vi "输入数据解析.vi"(0 "单个参数补充":dbl, 1 "从板号":dbl=1.0, 2 "主板二维码":string="BNET01", 3 "从板二维码":string="BNET01", 5 "主板引用":refnum<vi>, 7 "从板引用":refnum<vi>, 9 "主板选项":string="三级故障阀值", 11 "枚举":enum16{"主板", "从板"}(ring), 12 "快换":bool caption="快换写入") -> (4 "输出数组":dbl[][](array[numeric]), 6 "数组长度":dbl[](array[numeric]), 8 "循环次数":i32, 10 "命令":u32, 14 "名称":string[](array[string]), 15 "命令序号":u32[](array[numeric]))   [LabVIEW 2013] (continued)
                n3829 = Build Array(w9934) -> (w9935:dbl[])
              }
              frame 15 {
                # "极柱温度过高"
                n3830 = disable-structure shown="启用" {
                  disable-tunnel: w9945 -> [w9951 _]
                  disable-tunnel: [w9947 255 ("高字节1")] -> w9943
                  frame Disabled {
                    n3831 = Unbundle By Name(w9951) -> ("极柱温度过高"=w9950:dbl)
                    n3832 = call "输入分辨率计算-EV05.vi"("1字节?"=TRUE, "数值"=w9950, "偏移量"=-40.0, "分辨率"=1.0) -> ("高字节1"=w9947:dbl)  [unwired: 1 in, 6 out]
                  }
                  frame Enabled {
                  }
                }
                n3833 = Build Array(w9943) -> (w9944:i32[])
              }
              frame 16 {
                # "SOH过低"
                n3834 = disable-structure shown="启用" {
                  disable-tunnel: [w9968 w9976] -> w9955
                  disable-tunnel: w9954 -> [w9965 _]
                  disable-tunnel: [w9957 w9976] -> w9953
                  frame Disabled {
                    n3835 = Unbundle By Name(w9965) -> ("SOH过低"=w9964:dbl)
                    n3836 = call "输入分辨率计算-EV05.vi"("1字节?"=FALSE, "数值"=w9964, "偏移量"=0.0, "分辨率"=0.1) -> ("低字节"=w9966:dbl, "高字节1"=w9967:dbl)  [unwired: 1 in, 5 out]
                    n3837 = call "二进制解析-8.6.vi"("索引"=4, "数值"=w9967) -> ("低位子数组"=w9970:i32[])  [unwired: 3 out]
                    n3838 = call "二进制解析-8.6.vi"("索引"=4, "数值"=w9966) -> ("低位子数组"=w9959:i32[], "高位子数组"=w9969:i32[])  [unwired: 2 out]
                    n3839 = call "二进制解析-8.6.vi"("索引"=4, "数值"=0) -> ("低位子数组"=w9960:i32[])  [unwired: 3 out]
                    n3840 = Insert Into Array(array=w9970, new element=w9969) -> (w9963:i32[])  [unwired: 1 in]
                    n3841 = Insert Into Array(array=w9959, new element=w9960) -> (w9958:i32[])  [unwired: 1 in]
                    n3842 = call "数值二进制转十进制-8.6.vi"("子数组"=w9963) -> ("十进制数值"=w9968:i32)  [unwired: 4 out]
                    n3843 = call "数值二进制转十进制-8.6.vi"("子数组"=w9958) -> ("十进制数值"=w9957:i32)  [unwired: 4 out]
                  }
                  frame Enabled {
                    w9976 = 255 ("高字节1")
                  }
                }
                n3844 = Build Array(w9955, w9953) -> (w9956:i32[])
              }
            }
            n3845 = Insert Into Array(array=w9761, new element=w9762) -> (w9760:dbl[])  [unwired: 1 in]
          }
          n3846 = Build Array(w9757) -> (w9756:dbl[][])
          n3847 = Build Array("三级故障阀值") -> (w9747:string[])
        }
        frame "极柱温度过高" {
          n3848 = Unbundle By Name(w9982) -> ("一级故障"=w9983:refnum<vi>)
          n3849 = property class="Clust (严格)"(reference=w9983) -> ("Value"=w9981:T4)  [unwired: 1 in, 2 out]
          n3850 = for {
            N: 17 -> [_]
            tunnel: w9981 -> [w9993]
            shift-right: [w9990] -> w9987
            shift-left: dbl[] [] -> [w9991]
            i -> [w9994]
            n3851 = case shown="13" w9994 {
              tunnel: w9993 -> [w9995 w10006 w10017 w10027 w10037 w10047 w10059 w10071 w10083 w10095 w10107 w10119 w10133 w10154 w10166 w10175 w10184]
              tunnel: [w9996 w10007 w10018 w10028 w10038 w10049 w10061 w10073 w10085 w10097 w10109 w10120 w10142 w10157 w10165 w10174 w10186] -> w9992
              frame 0, Default {
                # "总电压过高"
                n3852 = disable-structure shown="启用" {
                  disable-tunnel: [w10002 w10005] -> w9998
                  disable-tunnel: [w10001 w10005] -> w9997
                  disable-tunnel: w9995 -> [w10000 _]
                  frame Disabled {
                    n3853 = Unbundle By Name(w10000) -> ("总电压过高"=w9999:dbl)
                    n3854 = call "输入分辨率计算-EV05.vi"("1字节?"=FALSE, "数值"=w9999, "分辨率"=0.1) -> ("低字节"=w10002:dbl, "高字节1"=w10001:dbl)  [unwired: 2 in, 5 out]
                  }
                  frame Enabled {
                    w10005 = 255 ("高字节1")
                  }
                }
                n3855 = Build Array(w9997, w9998) -> (w9996:i32[])
              }
              frame 1 {
                # "总电压过低"
                n3856 = disable-structure shown="启用" {
                  disable-tunnel: [w10013 w10016] -> w10009
                  disable-tunnel: [w10012 w10016] -> w10008
                  disable-tunnel: w10006 -> [w10011 _]
                  frame Disabled {
                    n3857 = Unbundle By Name(w10011) -> ("总电压过低"=w10010:dbl)
                    n3858 = call "输入分辨率计算-EV05.vi"("1字节?"=FALSE, "数值"=w10010, "分辨率"=0.1) -> ("低字节"=w10013:dbl, "高字节1"=w10012:dbl)  [unwired: 2 in, 5 out]
                  }
                  frame Enabled {
                    w10016 = 255 ("高字节1")
                  }
                }
                n3859 = Build Array(w10008, w10009) -> (w10007:i32[])
              }
              frame 2 {
                # "温度过高"
                n3860 = disable-structure shown="启用" {
                  disable-tunnel: [w10023 255 ("高字节1")] -> w10019
                  disable-tunnel: w10017 -> [w10021 _]
                  frame Disabled {
                    n3861 = Unbundle By Name(w10021) -> ("温度过高"=w10020:dbl)
                    n3862 = call "输入分辨率计算-EV05.vi"("1字节?"=TRUE, "数值"=w10020, "偏移量"=-40.0, "分辨率"=1.0) -> ("高字节1"=w10023:dbl)  [unwired: 1 in, 6 out]
                  }
                  frame Enabled {
                  }
                }
                n3863 = Build Array(w10019) -> (w10018:i32[])
              }
              frame 3 {
                # "温度过低"
                n3864 = disable-structure shown="启用" {
                  disable-tunnel: [w10033 255 ("高字节1")] -> w10029
                  disable-tunnel: w10027 -> [w10031 _]
                  frame Disabled {
                    n3865 = Unbundle By Name(w10031) -> ("温度过低"=w10030:dbl)
                    n3866 = call "输入分辨率计算-EV05.vi"("1字节?"=TRUE, "数值"=w10030, "偏移量"=-40.0, "分辨率"=1.0) -> ("高字节1"=w10033:dbl)  [unwired: 1 in, 6 out]
                  }
                  frame Enabled {
                  }
                }
                n3867 = Build Array(w10029) -> (w10028:i32[])
              }
              frame 4 {
                # "整组温度不均衡"
                n3868 = disable-structure shown="启用" {
                  disable-tunnel: [w10043 255 ("高字节1")] -> w10039
                  disable-tunnel: w10037 -> [w10041 _]
                  frame Disabled {
                    n3869 = Unbundle By Name(w10041) -> ("整组温度不均衡"=w10040:dbl)
                    n3870 = call "输入分辨率计算-EV05.vi"("1字节?"=TRUE, "数值"=w10040, "偏移量"=0.0, "分辨率"=1.0) -> ("高字节1"=w10043:dbl)  [unwired: 1 in, 6 out]
                  }
                  frame Enabled {
                  }
                }
                n3871 = Build Array(w10039) -> (w10038:i32[])
              }
              frame 5 {
                # "单组电压不均衡"
                n3872 = disable-structure shown="启用" {
                  disable-tunnel: [w10055 w10058] -> w10050
                  disable-tunnel: [w10053 w10058] -> w10048
                  disable-tunnel: w10047 -> [w10052 _]
                  frame Disabled {
                    n3873 = Unbundle By Name(w10052) -> ("单组电压不均衡"=w10051:dbl)
                    n3874 = call "输入分辨率计算-EV05.vi"("1字节?"=FALSE, "数值"=w10051, "偏移量"=0.0, "分辨率"=0.001) -> ("低字节"=w10053:dbl, "高字节1"=w10055:dbl)  [unwired: 1 in, 5 out]
                  }
                  frame Enabled {
                    w10058 = 255 ("高字节1")
                  }
                }
                n3875 = Build Array(w10050, w10048) -> (w10049:i32[])
              }
              frame 6 {
                # "整组电压不均衡"
                n3876 = disable-structure shown="启用" {
                  disable-tunnel: [w10067 w10070] -> w10062
                  disable-tunnel: [w10065 w10070] -> w10060
                  disable-tunnel: w10059 -> [w10064 _]
                  frame Disabled {
                    n3877 = Unbundle By Name(w10064) -> ("整组电压不均衡"=w10063:dbl)
                    n3878 = call "输入分辨率计算-EV05.vi"("1字节?"=FALSE, "数值"=w10063, "偏移量"=0.0, "分辨率"=0.001) -> ("低字节"=w10065:dbl, "高字节1"=w10067:dbl)  [unwired: 1 in, 5 out]
                  }
                  frame Enabled {
                    w10070 = 255 ("高字节1")
                  }
                }
                n3879 = Build Array(w10062, w10060) -> (w10061:i32[])
              }
              frame 7 {
                # "单体电压过高"
                n3880 = disable-structure shown="启用" {
                  disable-tunnel: [w10079 w10082] -> w10074
                  disable-tunnel: [w10077 w10082] -> w10072
                  disable-tunnel: w10071 -> [w10076 _]
                  frame Disabled {
                    n3881 = Unbundle By Name(w10076) -> ("单体电压过高"=w10075:dbl)
                    n3882 = call "输入分辨率计算-EV05.vi"("1字节?"=FALSE, "数值"=w10075, "偏移量"=0.0, "分辨率"=0.001) -> ("低字节"=w10077:dbl, "高字节1"=w10079:dbl)  [unwired: 1 in, 5 out]
                  }
                  frame Enabled {
                    w10082 = 255 ("高字节1")
                  }
                }
                n3883 = Build Array(w10074, w10072) -> (w10073:i32[])
              }
              frame 8 {
                # "单体电压过低"
                n3884 = disable-structure shown="启用" {
                  disable-tunnel: [w10091 w10094] -> w10086
                  disable-tunnel: [w10089 w10094] -> w10084
                  disable-tunnel: w10083 -> [w10088 _]
                  frame Disabled {
                    n3885 = Unbundle By Name(w10088) -> ("单体电压过低"=w10087:dbl)
                    n3886 = call "输入分辨率计算-EV05.vi"("1字节?"=FALSE, "数值"=w10087, "偏移量"=0.0, "分辨率"=0.001) -> ("低字节"=w10089:dbl, "高字节1"=w10091:dbl)  [unwired: 1 in, 5 out]
                  }
                  frame Enabled {
                    w10094 = 255 ("高字节1")
                  }
                }
                n3887 = Build Array(w10086, w10084) -> (w10085:i32[])
              }
              frame 9 {
                # "充电电流过高"
                n3888 = disable-structure shown="启用" {
                  disable-tunnel: [w10103 w10106] -> w10098
                  disable-tunnel: [w10101 w10106] -> w10096
                  disable-tunnel: w10095 -> [w10100 _]
                  frame Disabled {
                    n3889 = Unbundle By Name(w10100) -> ("充电电流过高"=w10099:dbl)
                    n3890 = call "输入分辨率计算-EV05.vi"("1字节?"=FALSE, "数值"=w10099, "偏移量"=-3000.0, "分辨率"=0.1) -> ("低字节"=w10101:dbl, "高字节1"=w10103:dbl)  [unwired: 1 in, 5 out]
                  }
                  frame Enabled {
                    w10106 = 255 ("高字节1")
                  }
                }
                n3891 = Build Array(w10098, w10096) -> (w10097:i32[])
              }
              frame 10 {
                # "放电电流过高"
                n3892 = disable-structure shown="启用" {
                  disable-tunnel: [w10115 w10118] -> w10110
                  disable-tunnel: [w10113 w10118] -> w10108
                  disable-tunnel: w10107 -> [w10112 _]
                  frame Disabled {
                    n3893 = Unbundle By Name(w10112) -> ("放电电流过高"=w10111:dbl)
                    n3894 = call "输入分辨率计算-EV05.vi"("1字节?"=FALSE, "数值"=w10111, "偏移量"=-3000.0, "分辨率"=0.1) -> ("低字节"=w10113:dbl, "高字节1"=w10115:dbl)  [unwired: 1 in, 5 out]
                  }
                  frame Enabled {
                    w10118 = 255 ("高字节1")
                  }
                }
                n3895 = Build Array(w10110, w10108) -> (w10109:i32[])
              }
              frame 11 {
                # "单组温度不均衡"
                n3896 = disable-structure shown="启用" {
                  disable-tunnel: [w10125 255 ("高字节1")] -> w10121
                  disable-tunnel: w10119 -> [w10123 _]
                  frame Disabled {
                    n3897 = Unbundle By Name(w10123) -> ("单组温度不均衡"=w10122:dbl)
                    n3898 = call "输入分辨率计算-EV05.vi"("1字节?"=TRUE, "数值"=w10122, "偏移量"=0.0, "分辨率"=1.0) -> ("高字节1"=w10125:dbl)  [unwired: 1 in, 6 out]
                  }
                  frame Enabled {
                  }
                }
                n3899 = Build Array(w10121) -> (w10120:i32[])
              }
              frame 12 {
                # "SOC过高"
                n3900 = Unbundle By Name(w10133) -> ("SOC过高"=w10132:dbl)
                n3901 = call "输入分辨率计算-EV05.vi"("1字节?"=FALSE, "数值"=w10132, "偏移量"=0.0, "分辨率"=0.1) -> ("低字节"=w10134:dbl, "高字节1"=w10135:dbl)  [unwired: 1 in, 5 out]
                n3902 = call "二进制解析-8.6.vi"("索引"=4, "数值"=w10135) -> ("低位子数组"=w10138:i32[])  [unwired: 3 out]
                n3903 = call "二进制解析-8.6.vi"("索引"=4, "数值"=w10134) -> ("低位子数组"=w10130:i32[], "高位子数组"=w10137:i32[])  [unwired: 2 out]
                n3904 = Insert Into Array(array=w10138, new element=w10137) -> (w10136:i32[])  [unwired: 1 in]
                n3905 = call "数值二进制转十进制-8.6.vi"("子数组"=w10136) -> ("十进制数值"=w10131:i32)  [unwired: 4 out]
                n3906 = disable-structure shown="启用" {
                  disable-tunnel: w10131 -> [w10146 _]
                  disable-tunnel: [w10146 255 ("高字节1")] -> w10129
                  disable-tunnel: w10130 -> [w10145 _]
                  disable-tunnel: [w10145 i32[] [] ("低位子数组 29")] -> _
                  frame Disabled {
                  }
                  frame Enabled {
                  }
                }
                n3907 = Build Array(w10129, w10129) -> (w10142:i32[])
              }
              frame 13 {
                # "SOC过低"
                n3908 = Unbundle By Name(w10154) -> ("SOC过低"=w10153:dbl)
                n3909 = call "输入分辨率计算-EV05.vi"("1字节?"=FALSE, "数值"=w10153, "偏移量"=0.0, "分辨率"=0.1) -> ("低字节"=w10151:dbl, "高字节1"=w10152:dbl)  [unwired: 1 in, 5 out]
                n3910 = call "二进制解析-8.6.vi"("索引"=4, "数值"=w10152) -> ("低位子数组"=w10150:i32[])  [unwired: 3 out]
                n3911 = disable-structure shown="启用" {
                  disable-tunnel: w10151 -> [w10161 _]
                  disable-tunnel: [w10161 255 ("高字节1")] -> w10149
                  disable-tunnel: w10150 -> [w10160 _]
                  disable-tunnel: [w10160 i32[] [] ("低位子数组")] -> _
                  frame Disabled {
                    (unwired) i32[] [] ("低位子数组 4")
                  }
                  frame Enabled {
                  }
                }
                n3912 = Build Array(w10149, w10149) -> (w10157:i32[])
              }
              frame 14 {
                # "内阻过大"
                n3913 = disable-structure shown="启用" {
                  disable-tunnel: w10166 -> [w10171 _]
                  disable-tunnel: [w10167 255 ("高字节1")] -> w10164
                  frame Disabled {
                    n3914 = Unbundle By Name(w10171) -> ("内阻过大"=w10170:dbl)
                    n3915 = call "输入分辨率计算-EV05.vi"("1字节?"=TRUE, "数值"=w10170, "分辨率"=0.1) -> ("高字节1"=w10167:dbl)  [unwired: 2 in, 6 out]
                  }
                  frame Enabled {
                  }
                }
                n3916 = Build Array(w10164) -> (w10165:i32[])
              }
              frame 15 {
                # "极柱温度过高"
                n3917 = disable-structure shown="启用" {
                  disable-tunnel: w10175 -> [w10181 _]
                  disable-tunnel: [w10177 255 ("高字节1")] -> w10173
                  frame Enabled {
                    n3918 = Unbundle By Name(w10181) -> ("极柱温度过高"=w10180:dbl)
                    n3919 = call "输入分辨率计算-EV05.vi"("1字节?"=TRUE, "数值"=w10180, "偏移量"=-40.0, "分辨率"=1.0) -> ("高字节1"=w10177:dbl)  [unwired: 1 in, 6 out]
                  }
                  frame Disabled {
                  }
                }
                n3920 = Build Array(w10173) -> (w10174:dbl[])
              }
              frame 16 {
                # "SOH过低"
                n3921 = disable-structure shown="启用" {
                  disable-tunnel: [w10198 w10206] -> w10185
                  disable-tunnel: w10184 -> [w10195 _]
                  disable-tunnel: [w10187 w10206] -> w10183
                  frame Disabled {
                    n3922 = Unbundle By Name(w10195) -> ("SOH过低"=w10194:dbl)
                    n3923 = call "输入分辨率计算-EV05.vi"("1字节?"=FALSE, "数值"=w10194, "偏移量"=0.0, "分辨率"=0.1) -> ("低字节"=w10196:dbl, "高字节1"=w10197:dbl)  [unwired: 1 in, 5 out]
                    n3924 = call "二进制解析-8.6.vi"("索引"=4, "数值"=w10197) -> ("低位子数组"=w10200:i32[])  [unwired: 3 out]
                    n3925 = call "二进制解析-8.6.vi"("索引"=4, "数值"=w10196) -> ("低位子数组"=w10189:i32[], "高位子数组"=w10199:i32[])  [unwired: 2 out]
                    n3926 = call "二进制解析-8.6.vi"("索引"=4, "数值"=0) -> ("低位子数组"=w10190:i32[])  [unwired: 3 out]
                    n3927 = Insert Into Array(array=w10200, new element=w10199) -> (w10193:i32[])  [unwired: 1 in]
                    n3928 = Insert Into Array(array=w10189, new element=w10190) -> (w10188:i32[])  [unwired: 1 in]
                    n3929 = call "数值二进制转十进制-8.6.vi"("子数组"=w10193) -> ("十进制数值"=w10198:i32)  [unwired: 4 out]
                    n3930 = call "数值二进制转十进制-8.6.vi"("子数组"=w10188) -> ("十进制数值"=w10187:i32)  [unwired: 4 out]
                  }
                  frame Enabled {
                    w10206 = 255 ("高字节1")
                  }
                }
                n3931 = Build Array(w10185, w10183) -> (w10186:i32[])
              }
            }
            n3932 = Insert Into Array(array=w9991, new element=w9992) -> (w9990:dbl[])  [unwired: 1 in]
          }
          n3933 = Build Array(w9987) -> (w9986:dbl[][])
          n3934 = Build Array("一级故障阀值") -> (w9977:string[])
        }
        frame "极柱温度过高(2)" {
          n3935 = Unbundle By Name(w10212) -> ("一级故障 2"=w10213:refnum<vi>)
          n3936 = property class="Clust (严格)"(reference=w10213) -> ("Value"=w10211:T4)  [unwired: 1 in, 2 out]
          n3937 = for {
            N: 17 -> [_]
            tunnel: w10211 -> [w10223]
            shift-right: [w10220] -> w10217
            shift-left: dbl[] [] -> [w10221]
            i -> [w10224]
            n3938 = case shown="13" w10224 {
              tunnel: w10223 -> [w10225 w10236 w10247 w10257 w10267 w10277 w10289 w10301 w10313 w10325 w10337 w10349 w10363 w10384 w10396 w10405 w10414]
              tunnel: [w10226 w10237 w10248 w10258 w10268 w10279 w10291 w10303 w10315 w10327 w10339 w10350 w10372 w10387 w10395 w10404 w10416] -> w10222
              frame 0, Default {
                # "总电压过高"
                n3939 = disable-structure shown="启用" {
                  disable-tunnel: [w10232 w10235] -> w10228
                  disable-tunnel: [w10231 w10235] -> w10227
                  disable-tunnel: w10225 -> [w10230 _]
                  frame Disabled {
                    n3940 = Unbundle By Name(w10230) -> ("总电压过高"=w10229:dbl)
                    n3941 = call "输入分辨率计算-EV05.vi"("1字节?"=FALSE, "数值"=w10229, "分辨率"=0.1) -> ("低字节"=w10232:dbl, "高字节1"=w10231:dbl)  [unwired: 2 in, 5 out]
                  }
                  frame Enabled {
                    w10235 = 255 ("高字节1")
                  }
                }
                n3942 = Build Array(w10227, w10228) -> (w10226:i32[])
              }
              frame 1 {
                # "总电压过低"
                n3943 = disable-structure shown="启用" {
                  disable-tunnel: [w10243 w10246] -> w10239
                  disable-tunnel: [w10242 w10246] -> w10238
                  disable-tunnel: w10236 -> [w10241 _]
                  frame Disabled {
                    n3944 = Unbundle By Name(w10241) -> ("总电压过低"=w10240:dbl)
                    n3945 = call "输入分辨率计算-EV05.vi"("1字节?"=FALSE, "数值"=w10240, "分辨率"=0.1) -> ("低字节"=w10243:dbl, "高字节1"=w10242:dbl)  [unwired: 2 in, 5 out]
                  }
                  frame Enabled {
                    w10246 = 255 ("高字节1")
                  }
                }
                n3946 = Build Array(w10238, w10239) -> (w10237:i32[])
              }
              frame 2 {
                # "温度过高"
                n3947 = disable-structure shown="启用" {
                  disable-tunnel: [w10253 255 ("高字节1")] -> w10249
                  disable-tunnel: w10247 -> [w10251 _]
                  frame Disabled {
                    n3948 = Unbundle By Name(w10251) -> ("温度过高"=w10250:dbl)
                    n3949 = call "输入分辨率计算-EV05.vi"("1字节?"=TRUE, "数值"=w10250, "偏移量"=-40.0, "分辨率"=1.0) -> ("高字节1"=w10253:dbl)  [unwired: 1 in, 6 out]
                  }
                  frame Enabled {
                  }
                }
                n3950 = Build Array(w10249) -> (w10248:i32[])
              }
              frame 3 {
                # "温度过低"
                n3951 = disable-structure shown="启用" {
                  disable-tunnel: [w10263 255 ("高字节1")] -> w10259
                  disable-tunnel: w10257 -> [w10261 _]
                  frame Disabled {
                    n3952 = Unbundle By Name(w10261) -> ("温度过低"=w10260:dbl)
                    n3953 = call "输入分辨率计算-EV05.vi"("1字节?"=TRUE, "数值"=w10260, "偏移量"=-40.0, "分辨率"=1.0) -> ("高字节1"=w10263:dbl)  [unwired: 1 in, 6 out]
                  }
                  frame Enabled {
                  }
                }
                n3954 = Build Array(w10259) -> (w10258:i32[])
              }
              frame 4 {
                # "整组温度不均衡"
                n3955 = disable-structure shown="启用" {
                  disable-tunnel: [w10273 255 ("高字节1")] -> w10269
                  disable-tunnel: w10267 -> [w10271 _]
                  frame Disabled {
                    n3956 = Unbundle By Name(w10271) -> ("整组温度不均衡"=w10270:dbl)
                    n3957 = call "输入分辨率计算-EV05.vi"("1字节?"=TRUE, "数值"=w10270, "偏移量"=0.0, "分辨率"=1.0) -> ("高字节1"=w10273:dbl)  [unwired: 1 in, 6 out]
                  }
                  frame Enabled {
                  }
                }
                n3958 = Build Array(w10269) -> (w10268:i32[])
              }
              frame 5 {
                # "单组电压不均衡"
                n3959 = disable-structure shown="启用" {
                  disable-tunnel: [w10285 w10288] -> w10280
                  disable-tunnel: [w10283 w10288] -> w10278
                  disable-tunnel: w10277 -> [w10282 _]
                  frame Disabled {
                    n3960 = Unbundle By Name(w10282) -> ("单组电压不均衡"=w10281:dbl)
                    n3961 = call "输入分辨率计算-EV05.vi"("1字节?"=FALSE, "数值"=w10281, "偏移量"=0.0, "分辨率"=0.001) -> ("低字节"=w10283:dbl, "高字节1"=w10285:dbl)  [unwired: 1 in, 5 out]
                  }
                  frame Enabled {
                    w10288 = 255 ("高字节1")
                  }
                }
                n3962 = Build Array(w10280, w10278) -> (w10279:i32[])
              }
              frame 6 {
                # "整组电压不均衡"
                n3963 = disable-structure shown="启用" {
                  disable-tunnel: [w10297 w10300] -> w10292
                  disable-tunnel: [w10295 w10300] -> w10290
                  disable-tunnel: w10289 -> [w10294 _]
                  frame Disabled {
                    n3964 = Unbundle By Name(w10294) -> ("整组电压不均衡"=w10293:dbl)
                    n3965 = call "输入分辨率计算-EV05.vi"("1字节?"=FALSE, "数值"=w10293, "偏移量"=0.0, "分辨率"=0.001) -> ("低字节"=w10295:dbl, "高字节1"=w10297:dbl)  [unwired: 1 in, 5 out]
                  }
                  frame Enabled {
                    w10300 = 255 ("高字节1")
                  }
                }
                n3966 = Build Array(w10292, w10290) -> (w10291:i32[])
              }
              frame 7 {
                # "单体电压过高"
                n3967 = disable-structure shown="启用" {
                  disable-tunnel: [w10309 w10312] -> w10304
                  disable-tunnel: [w10307 w10312] -> w10302
                  disable-tunnel: w10301 -> [w10306 _]
                  frame Disabled {
                    n3968 = Unbundle By Name(w10306) -> ("单体电压过高"=w10305:dbl)
                    n3969 = call "输入分辨率计算-EV05.vi"("1字节?"=FALSE, "数值"=w10305, "偏移量"=0.0, "分辨率"=0.001) -> ("低字节"=w10307:dbl, "高字节1"=w10309:dbl)  [unwired: 1 in, 5 out]
                  }
                  frame Enabled {
                    w10312 = 255 ("高字节1")
                  }
                }
                n3970 = Build Array(w10304, w10302) -> (w10303:i32[])
              }
              frame 8 {
                # "单体电压过低"
                n3971 = disable-structure shown="启用" {
                  disable-tunnel: [w10321 w10324] -> w10316
                  disable-tunnel: [w10319 w10324] -> w10314
                  disable-tunnel: w10313 -> [w10318 _]
                  frame Disabled {
                    n3972 = Unbundle By Name(w10318) -> ("单体电压过低"=w10317:dbl)
                    n3973 = call "输入分辨率计算-EV05.vi"("1字节?"=FALSE, "数值"=w10317, "偏移量"=0.0, "分辨率"=0.001) -> ("低字节"=w10319:dbl, "高字节1"=w10321:dbl)  [unwired: 1 in, 5 out]
                  }
                  frame Enabled {
                    w10324 = 255 ("高字节1")
                  }
                }
                n3974 = Build Array(w10316, w10314) -> (w10315:i32[])
              }
              frame 9 {
                # "充电电流过高"
                n3975 = disable-structure shown="启用" {
                  disable-tunnel: [w10333 w10336] -> w10328
                  disable-tunnel: [w10331 w10336] -> w10326
                  disable-tunnel: w10325 -> [w10330 _]
                  frame Disabled {
                    n3976 = Unbundle By Name(w10330) -> ("充电电流过高"=w10329:dbl)
                    n3977 = call "输入分辨率计算-EV05.vi"("1字节?"=FALSE, "数值"=w10329, "偏移量"=-3000.0, "分辨率"=0.1) -> ("低字节"=w10331:dbl, "高字节1"=w10333:dbl)  [unwired: 1 in, 5 out]
                  }
                  frame Enabled {
                    w10336 = 255 ("高字节1")
                  }
                }
                n3978 = Build Array(w10328, w10326) -> (w10327:i32[])
              }
              frame 10 {
                # "放电电流过高"
                n3979 = disable-structure shown="启用" {
                  disable-tunnel: [w10345 w10348] -> w10340
                  disable-tunnel: [w10343 w10348] -> w10338
                  disable-tunnel: w10337 -> [w10342 _]
                  frame Disabled {
                    n3980 = Unbundle By Name(w10342) -> ("放电电流过高"=w10341:dbl)
                    n3981 = call "输入分辨率计算-EV05.vi"("1字节?"=FALSE, "数值"=w10341, "偏移量"=-3000.0, "分辨率"=0.1) -> ("低字节"=w10343:dbl, "高字节1"=w10345:dbl)  [unwired: 1 in, 5 out]
                  }
                  frame Enabled {
                    w10348 = 255 ("高字节1")
                  }
                }
                n3982 = Build Array(w10340, w10338) -> (w10339:i32[])
              }
              frame 11 {
                # "单组温度不均衡"
                n3983 = disable-structure shown="启用" {
                  disable-tunnel: [w10355 255 ("高字节1")] -> w10351
                  disable-tunnel: w10349 -> [w10353 _]
                  frame Disabled {
                    n3984 = Unbundle By Name(w10353) -> ("单组温度不均衡"=w10352:dbl)
                    n3985 = call "输入分辨率计算-EV05.vi"("1字节?"=TRUE, "数值"=w10352, "偏移量"=0.0, "分辨率"=1.0) -> ("高字节1"=w10355:dbl)  [unwired: 1 in, 6 out]
                  }
                  frame Enabled {
                  }
                }
                n3986 = Build Array(w10351) -> (w10350:i32[])
              }
              frame 12 {
                # "SOC过高"
                n3987 = Unbundle By Name(w10363) -> ("SOC过高"=w10362:dbl)
                n3988 = call "输入分辨率计算-EV05.vi"("1字节?"=FALSE, "数值"=w10362, "偏移量"=0.0, "分辨率"=0.1) -> ("低字节"=w10364:dbl, "高字节1"=w10365:dbl)  [unwired: 1 in, 5 out]
                n3989 = call "二进制解析-8.6.vi"("索引"=4, "数值"=w10365) -> ("低位子数组"=w10368:i32[])  [unwired: 3 out]
                n3990 = call "二进制解析-8.6.vi"("索引"=4, "数值"=w10364) -> ("低位子数组"=w10360:i32[], "高位子数组"=w10367:i32[])  [unwired: 2 out]
                n3991 = Insert Into Array(array=w10368, new element=w10367) -> (w10366:i32[])  [unwired: 1 in]
                n3992 = call "数值二进制转十进制-8.6.vi"("子数组"=w10366) -> ("十进制数值"=w10361:i32)  [unwired: 4 out]
                n3993 = disable-structure shown="启用" {
                  disable-tunnel: w10361 -> [w10376 _]
                  disable-tunnel: [w10376 255 ("高字节1")] -> w10359
                  disable-tunnel: w10360 -> [w10375 _]
                  disable-tunnel: [w10375 i32[] [] ("低位子数组 29")] -> _
                  frame Disabled {
                  }
                  frame Enabled {
                  }
                }
                n3994 = Build Array(w10359, w10359) -> (w10372:i32[])
              }
              frame 13 {
                # "SOC过低"
                n3995 = Unbundle By Name(w10384) -> ("SOC过低"=w10383:dbl)
                n3996 = call "输入分辨率计算-EV05.vi"("1字节?"=FALSE, "数值"=w10383, "偏移量"=0.0, "分辨率"=0.1) -> ("低字节"=w10381:dbl, "高字节1"=w10382:dbl)  [unwired: 1 in, 5 out]
                n3997 = call "二进制解析-8.6.vi"("索引"=4, "数值"=w10382) -> ("低位子数组"=w10380:i32[])  [unwired: 3 out]
                n3998 = disable-structure shown="启用" {
                  disable-tunnel: w10381 -> [w10391 _]
                  disable-tunnel: [w10391 255 ("高字节1")] -> w10379
                  disable-tunnel: w10380 -> [w10390 _]
                  disable-tunnel: [w10390 i32[] [] ("低位子数组")] -> _
                  frame Disabled {
                    (unwired) i32[] [] ("低位子数组 4")
                  }
                  frame Enabled {
                  }
                }
                n3999 = Build Array(w10379, w10379) -> (w10387:i32[])
              }
              frame 14 {
                # "内阻过大"
                n4000 = disable-structure shown="启用" {
                  disable-tunnel: w10396 -> [w10401 _]
                  disable-tunnel: [w10397 255 ("高字节1")] -> w10394
                  frame Disabled {
                    n4001 = Unbundle By Name(w10401) -> ("内阻过大"=w10400:dbl)
                    n4002 = call "输入分辨率计算-EV05.vi"("1字节?"=TRUE, "数值"=w10400, "分辨率"=0.1) -> ("高字节1"=w10397:dbl)  [unwired: 2 in, 6 out]
                  }
                  frame Enabled {
                  }
                }
                n4003 = Build Array(w10394) -> (w10395:i32[])
              }
              frame 15 {
                # "极柱温度过高"
                n4004 = disable-structure shown="启用" {
                  disable-tunnel: w10405 -> [w10411 _]
                  disable-tunnel: [w10407 255 ("高字节1")] -> w10403
                  frame Enabled {
                    n4005 = Unbundle By Name(w10411) -> ("极柱温度过高"=w10410:dbl)
                    n4006 = call "输入分辨率计算-EV05.vi"("1字节?"=TRUE, "数值"=w10410, "偏移量"=-40.0, "分辨率"=1.0) -> ("高字节1"=w10407:dbl)  [unwired: 1 in, 6 out]
                  }
                  frame Disabled {
                  }
                }
                n4007 = Build Array(w10403) -> (w10404:dbl[])
              }
              frame 16 {
                # "SOH过低"
                n4008 = disable-structure shown="启用" {
                  disable-tunnel: [w10428 w10436] -> w10415
                  disable-tunnel: w10414 -> [w10425 _]
                  disable-tunnel: [w10417 w10436] -> w10413
                  frame Disabled {
                    n4009 = Unbundle By Name(w10425) -> ("SOH过低"=w10424:dbl)
                    n4010 = call "输入分辨率计算-EV05.vi"("1字节?"=FALSE, "数值"=w10424, "偏移量"=0.0, "分辨率"=0.1) -> ("低字节"=w10426:dbl, "高字节1"=w10427:dbl)  [unwired: 1 in, 5 out]
                    n4011 = call "二进制解析-8.6.vi"("索引"=4, "数值"=w10427) -> ("低位子数组"=w10430:i32[])  [unwired: 3 out]
                    n4012 = call "二进制解析-8.6.vi"("索引"=4, "数值"=w10426) -> ("低位子数组"=w10419:i32[], "高位子数组"=w10429:i32[])  [unwired: 2 out]
                    n4013 = call "二进制解析-8.6.vi"("索引"=4, "数值"=0) -> ("低位子数组"=w10420:i32[])  [unwired: 3 out]
                    n4014 = Insert Into Array(array=w10430, new element=w10429) -> (w10423:i32[])  [unwired: 1 in]
                    n4015 = Insert Into Array(array=w10419, new element=w10420) -> (w10418:i32[])  [unwired: 1 in]
                    n4016 = call "数值二进制转十进制-8.6.vi"("子数组"=w10423) -> ("十进制数值"=w10428:i32)  [unwired: 4 out]
                    n4017 = call "数值二进制转十进制-8.6.vi"("子数组"=w10418) -> ("十进制数值"=w10417:i32)  [unwired: 4 out]
                  }
                  frame Enabled {
                    w10436 = 255 ("高字节1")
                  }
                }
                n4018 = Build Array(w10415, w10413) -> (w10416:i32[])
              }
            }
            n4019 = Insert Into Array(array=w10221, new element=w10222) -> (w10220:dbl[])  [unwired: 1 in]
          }
          n4020 = Build Array(w10217) -> (w10216:dbl[][])
          n4021 = Build Array("二级故障阀值") -> (w10207:string[])
        }
        frame "极柱温度过高(3)" {
          n4022 = Unbundle By Name(w10442) -> ("一级故障 3"=w10443:refnum<vi>)
          n4023 = property class="Clust (严格)"(reference=w10443) -> ("Value"=w10441:T4)  [unwired: 1 in, 2 out]
          n4024 = for {
            N: 17 -> [_]
            tunnel: w10441 -> [w10453]
            shift-right: [w10450] -> w10447
            shift-left: dbl[] [] -> [w10451]
            i -> [w10454]
            n4025 = case shown="13" w10454 {
              tunnel: w10453 -> [w10455 w10466 w10477 w10487 w10497 w10507 w10519 w10531 w10543 w10555 w10567 w10579 w10593 w10614 w10626 w10635 w10644]
              tunnel: [w10456 w10467 w10478 w10488 w10498 w10509 w10521 w10533 w10545 w10557 w10569 w10580 w10602 w10617 w10625 w10634 w10646] -> w10452
              frame 0, Default {
                # "总电压过高"
                n4026 = disable-structure shown="启用" {
                  disable-tunnel: [w10462 w10465] -> w10458
                  disable-tunnel: [w10461 w10465] -> w10457
                  disable-tunnel: w10455 -> [w10460 _]
                  frame Disabled {
                    n4027 = Unbundle By Name(w10460) -> ("总电压过高"=w10459:dbl)
                    n4028 = call "输入分辨率计算-EV05.vi"("1字节?"=FALSE, "数值"=w10459, "分辨率"=0.1) -> ("低字节"=w10462:dbl, "高字节1"=w10461:dbl)  [unwired: 2 in, 5 out]
                  }
                  frame Enabled {
                    w10465 = 255 ("高字节1")
                  }
                }
                n4029 = Build Array(w10457, w10458) -> (w10456:i32[])
              }
              frame 1 {
                # "总电压过低"
                n4030 = disable-structure shown="启用" {
                  disable-tunnel: [w10473 w10476] -> w10469
                  disable-tunnel: [w10472 w10476] -> w10468
                  disable-tunnel: w10466 -> [w10471 _]
                  frame Disabled {
                    n4031 = Unbundle By Name(w10471) -> ("总电压过低"=w10470:dbl)
                    n4032 = call "输入分辨率计算-EV05.vi"("1字节?"=FALSE, "数值"=w10470, "分辨率"=0.1) -> ("低字节"=w10473:dbl, "高字节1"=w10472:dbl)  [unwired: 2 in, 5 out]
                  }
                  frame Enabled {
                    w10476 = 255 ("高字节1")
                  }
                }
                n4033 = Build Array(w10468, w10469) -> (w10467:i32[])
              }
              frame 2 {
                # "温度过高"
                n4034 = disable-structure shown="启用" {
                  disable-tunnel: [w10483 255 ("高字节1")] -> w10479
                  disable-tunnel: w10477 -> [w10481 _]
                  frame Disabled {
                    n4035 = Unbundle By Name(w10481) -> ("温度过高"=w10480:dbl)
                    n4036 = call "输入分辨率计算-EV05.vi"("1字节?"=TRUE, "数值"=w10480, "偏移量"=-40.0, "分辨率"=1.0) -> ("高字节1"=w10483:dbl)  [unwired: 1 in, 6 out]
                  }
                  frame Enabled {
                  }
                }
                n4037 = Build Array(w10479) -> (w10478:i32[])
              }
              frame 3 {
                # "温度过低"
                n4038 = disable-structure shown="启用" {
                  disable-tunnel: [w10493 255 ("高字节1")] -> w10489
                  disable-tunnel: w10487 -> [w10491 _]
                  frame Disabled {
                    n4039 = Unbundle By Name(w10491) -> ("温度过低"=w10490:dbl)
                    n4040 = call "输入分辨率计算-EV05.vi"("1字节?"=TRUE, "数值"=w10490, "偏移量"=-40.0, "分辨率"=1.0) -> ("高字节1"=w10493:dbl)  [unwired: 1 in, 6 out]
                  }
                  frame Enabled {
                  }
                }
                n4041 = Build Array(w10489) -> (w10488:i32[])
              }
              frame 4 {
                # "整组温度不均衡"
                n4042 = disable-structure shown="启用" {
                  disable-tunnel: [w10503 255 ("高字节1")] -> w10499
                  disable-tunnel: w10497 -> [w10501 _]
                  frame Disabled {
                    n4043 = Unbundle By Name(w10501) -> ("整组温度不均衡"=w10500:dbl)
                    n4044 = call "输入分辨率计算-EV05.vi"("1字节?"=TRUE, "数值"=w10500, "偏移量"=0.0, "分辨率"=1.0) -> ("高字节1"=w10503:dbl)  [unwired: 1 in, 6 out]
                  }
                  frame Enabled {
                  }
                }
                n4045 = Build Array(w10499) -> (w10498:i32[])
              }
              frame 5 {
                # "单组电压不均衡"
                n4046 = disable-structure shown="启用" {
                  disable-tunnel: [w10515 w10518] -> w10510
                  disable-tunnel: [w10513 w10518] -> w10508
                  disable-tunnel: w10507 -> [w10512 _]
                  frame Disabled {
                    n4047 = Unbundle By Name(w10512) -> ("单组电压不均衡"=w10511:dbl)
                    n4048 = call "输入分辨率计算-EV05.vi"("1字节?"=FALSE, "数值"=w10511, "偏移量"=0.0, "分辨率"=0.001) -> ("低字节"=w10513:dbl, "高字节1"=w10515:dbl)  [unwired: 1 in, 5 out]
                  }
                  frame Enabled {
                    w10518 = 255 ("高字节1")
                  }
                }
                n4049 = Build Array(w10510, w10508) -> (w10509:i32[])
              }
              frame 6 {
                # "整组电压不均衡"
                n4050 = disable-structure shown="启用" {
                  disable-tunnel: [w10527 w10530] -> w10522
                  disable-tunnel: [w10525 w10530] -> w10520
                  disable-tunnel: w10519 -> [w10524 _]
                  frame Disabled {
                    n4051 = Unbundle By Name(w10524) -> ("整组电压不均衡"=w10523:dbl)
                    n4052 = call "输入分辨率计算-EV05.vi"("1字节?"=FALSE, "数值"=w10523, "偏移量"=0.0, "分辨率"=0.001) -> ("低字节"=w10525:dbl, "高字节1"=w10527:dbl)  [unwired: 1 in, 5 out]
                  }
                  frame Enabled {
                    w10530 = 255 ("高字节1")
                  }
                }
                n4053 = Build Array(w10522, w10520) -> (w10521:i32[])
              }
              frame 7 {
                # "单体电压过高"
                n4054 = disable-structure shown="启用" {
                  disable-tunnel: [w10539 w10542] -> w10534
                  disable-tunnel: [w10537 w10542] -> w10532
                  disable-tunnel: w10531 -> [w10536 _]
                  frame Disabled {
                    n4055 = Unbundle By Name(w10536) -> ("单体电压过高"=w10535:dbl)
                    n4056 = call "输入分辨率计算-EV05.vi"("1字节?"=FALSE, "数值"=w10535, "偏移量"=0.0, "分辨率"=0.001) -> ("低字节"=w10537:dbl, "高字节1"=w10539:dbl)  [unwired: 1 in, 5 out]
                  }
                  frame Enabled {
                    w10542 = 255 ("高字节1")
                  }
                }
                n4057 = Build Array(w10534, w10532) -> (w10533:i32[])
              }
              frame 8 {
                # "单体电压过低"
                n4058 = disable-structure shown="启用" {
                  disable-tunnel: [w10551 w10554] -> w10546
                  disable-tunnel: [w10549 w10554] -> w10544
                  disable-tunnel: w10543 -> [w10548 _]
                  frame Disabled {
                    n4059 = Unbundle By Name(w10548) -> ("单体电压过低"=w10547:dbl)
                    n4060 = call "输入分辨率计算-EV05.vi"("1字节?"=FALSE, "数值"=w10547, "偏移量"=0.0, "分辨率"=0.001) -> ("低字节"=w10549:dbl, "高字节1"=w10551:dbl)  [unwired: 1 in, 5 out]
                  }
                  frame Enabled {
                    w10554 = 255 ("高字节1")
                  }
                }
                n4061 = Build Array(w10546, w10544) -> (w10545:i32[])
              }
              frame 9 {
                # "充电电流过高"
                n4062 = disable-structure shown="启用" {
                  disable-tunnel: [w10563 w10566] -> w10558
                  disable-tunnel: [w10561 w10566] -> w10556
                  disable-tunnel: w10555 -> [w10560 _]
                  frame Disabled {
                    n4063 = Unbundle By Name(w10560) -> ("充电电流过高"=w10559:dbl)
                    n4064 = call "输入分辨率计算-EV05.vi"("1字节?"=FALSE, "数值"=w10559, "偏移量"=-3000.0, "分辨率"=0.1) -> ("低字节"=w10561:dbl, "高字节1"=w10563:dbl)  [unwired: 1 in, 5 out]
                  }
                  frame Enabled {
                    w10566 = 255 ("高字节1")
                  }
                }
                n4065 = Build Array(w10558, w10556) -> (w10557:i32[])
              }
              frame 10 {
                # "放电电流过高"
                n4066 = disable-structure shown="启用" {
                  disable-tunnel: [w10575 w10578] -> w10570
                  disable-tunnel: [w10573 w10578] -> w10568
                  disable-tunnel: w10567 -> [w10572 _]
                  frame Disabled {
                    n4067 = Unbundle By Name(w10572) -> ("放电电流过高"=w10571:dbl)
                    n4068 = call "输入分辨率计算-EV05.vi"("1字节?"=FALSE, "数值"=w10571, "偏移量"=-3000.0, "分辨率"=0.1) -> ("低字节"=w10573:dbl, "高字节1"=w10575:dbl)  [unwired: 1 in, 5 out]
                  }
                  frame Enabled {
                    w10578 = 255 ("高字节1")
                  }
                }
                n4069 = Build Array(w10570, w10568) -> (w10569:i32[])
              }
              frame 11 {
                # "单组温度不均衡"
                n4070 = disable-structure shown="启用" {
                  disable-tunnel: [w10585 255 ("高字节1")] -> w10581
                  disable-tunnel: w10579 -> [w10583 _]
                  frame Disabled {
                    n4071 = Unbundle By Name(w10583) -> ("单组温度不均衡"=w10582:dbl)
                    n4072 = call "输入分辨率计算-EV05.vi"("1字节?"=TRUE, "数值"=w10582, "偏移量"=0.0, "分辨率"=1.0) -> ("高字节1"=w10585:dbl)  [unwired: 1 in, 6 out]
                  }
                  frame Enabled {
                  }
                }
                n4073 = Build Array(w10581) -> (w10580:i32[])
              }
              frame 12 {
                # "SOC过高"
                n4074 = Unbundle By Name(w10593) -> ("SOC过高"=w10592:dbl)
                n4075 = call "输入分辨率计算-EV05.vi"("1字节?"=FALSE, "数值"=w10592, "偏移量"=0.0, "分辨率"=0.1) -> ("低字节"=w10594:dbl, "高字节1"=w10595:dbl)  [unwired: 1 in, 5 out]
                n4076 = call "二进制解析-8.6.vi"("索引"=4, "数值"=w10595) -> ("低位子数组"=w10598:i32[])  [unwired: 3 out]
                n4077 = call "二进制解析-8.6.vi"("索引"=4, "数值"=w10594) -> ("低位子数组"=w10590:i32[], "高位子数组"=w10597:i32[])  [unwired: 2 out]
                n4078 = Insert Into Array(array=w10598, new element=w10597) -> (w10596:i32[])  [unwired: 1 in]
                n4079 = call "数值二进制转十进制-8.6.vi"("子数组"=w10596) -> ("十进制数值"=w10591:i32)  [unwired: 4 out]
                n4080 = disable-structure shown="启用" {
                  disable-tunnel: w10591 -> [w10606 _]
                  disable-tunnel: [w10606 255 ("高字节1")] -> w10589
                  disable-tunnel: w10590 -> [w10605 _]
                  disable-tunnel: [w10605 i32[] [] ("低位子数组 29")] -> _
                  frame Disabled {
                  }
                  frame Enabled {
                  }
                }
                n4081 = Build Array(w10589, w10589) -> (w10602:i32[])
              }
              frame 13 {
                # "SOC过低"
                n4082 = Unbundle By Name(w10614) -> ("SOC过低"=w10613:dbl)
                n4083 = call "输入分辨率计算-EV05.vi"("1字节?"=FALSE, "数值"=w10613, "偏移量"=0.0, "分辨率"=0.1) -> ("低字节"=w10611:dbl, "高字节1"=w10612:dbl)  [unwired: 1 in, 5 out]
                n4084 = call "二进制解析-8.6.vi"("索引"=4, "数值"=w10612) -> ("低位子数组"=w10610:i32[])  [unwired: 3 out]
                n4085 = disable-structure shown="启用" {
                  disable-tunnel: w10611 -> [w10621 _]
                  disable-tunnel: [w10621 255 ("高字节1")] -> w10609
                  disable-tunnel: w10610 -> [w10620 _]
                  disable-tunnel: [w10620 i32[] [] ("低位子数组")] -> _
                  frame Disabled {
                    (unwired) i32[] [] ("低位子数组 4")
                  }
                  frame Enabled {
                  }
                }
                n4086 = Build Array(w10609, w10609) -> (w10617:i32[])
              }
              frame 14 {
                # "内阻过大"
                n4087 = disable-structure shown="启用" {
                  disable-tunnel: w10626 -> [w10631 _]
                  disable-tunnel: [w10627 255 ("高字节1")] -> w10624
                  frame Disabled {
                    n4088 = Unbundle By Name(w10631) -> ("内阻过大"=w10630:dbl)
                    n4089 = call "输入分辨率计算-EV05.vi"("1字节?"=TRUE, "数值"=w10630, "分辨率"=0.1) -> ("高字节1"=w10627:dbl)  [unwired: 2 in, 6 out]
                  }
                  frame Enabled {
                  }
                }
                n4090 = Build Array(w10624) -> (w10625:i32[])
              }
              frame 15 {
                # "极柱温度过高"
                n4091 = disable-structure shown="启用" {
                  disable-tunnel: w10635 -> [w10641 _]
                  disable-tunnel: [w10637 255 ("高字节1")] -> w10633
                  frame Enabled {
                    n4092 = Unbundle By Name(w10641) -> ("极柱温度过高"=w10640:dbl)
                    n4093 = call "输入分辨率计算-EV05.vi"("1字节?"=TRUE, "数值"=w10640, "偏移量"=-40.0, "分辨率"=1.0) -> ("高字节1"=w10637:dbl)  [unwired: 1 in, 6 out]
                  }
                  frame Disabled {
                  }
                }
                n4094 = Build Array(w10633) -> (w10634:dbl[])
              }
              frame 16 {
                # "SOH过低"
                n4095 = disable-structure shown="启用" {
                  disable-tunnel: [w10658 w10666] -> w10645
                  disable-tunnel: w10644 -> [w10655 _]
                  disable-tunnel: [w10647 w10666] -> w10643
                  frame Disabled {
                    n4096 = Unbundle By Name(w10655) -> ("SOH过低"=w10654:dbl)
                    n4097 = call "输入分辨率计算-EV05.vi"("1字节?"=FALSE, "数值"=w10654, "偏移量"=0.0, "分辨率"=0.1) -> ("低字节"=w10656:dbl, "高字节1"=w10657:dbl)  [unwired: 1 in, 5 out]
                    n4098 = call "二进制解析-8.6.vi"("索引"=4, "数值"=w10657) -> ("低位子数组"=w10660:i32[])  [unwired: 3 out]
                    n4099 = call "二进制解析-8.6.vi"("索引"=4, "数值"=w10656) -> ("低位子数组"=w10649:i32[], "高位子数组"=w10659:i32[])  [unwired: 2 out]
                    n4100 = call "二进制解析-8.6.vi"("索引"=4, "数值"=0) -> ("低位子数组"=w10650:i32[])  [unwired: 3 out]
                    n4101 = Insert Into Array(array=w10660, new element=w10659) -> (w10653:i32[])  [unwired: 1 in]
                    n4102 = Insert Into Array(array=w10649, new element=w10650) -> (w10648:i32[])  [unwired: 1 in]
                    n4103 = call "数值二进制转十进制-8.6.vi"("子数组"=w10653) -> ("十进制数值"=w10658:i32)  [unwired: 4 out]
                    n4104 = call "数值二进制转十进制-8.6.vi"("子数组"=w10648) -> ("十进制数值"=w10647:i32)  [unwired: 4 out]
                  }
                  frame Enabled {
                    w10666 = 255 ("高字节1")
                  }
                }
                n4105 = Build Array(w10645, w10643) -> (w10646:i32[])
              }
            }
            n4106 = Insert Into Array(array=w10451, new element=w10452) -> (w10450:dbl[])  [unwired: 1 in]
          }
          n4107 = Build Array(w10447) -> (w10446:dbl[][])
          n4108 = Build Array("三级故障阀值") -> (w10437:string[])
        }
        frame "SOH过低" {
          n4109 = Unbundle By Name(w10672) -> ("一级故障"=w10673:refnum<vi>)
          n4110 = property class="Clust (严格)"(reference=w10673) -> ("Value"=w10671:T4)  [unwired: 1 in, 2 out]
          n4111 = for {
            N: 17 -> [_]
            tunnel: w10671 -> [w10683]
            shift-right: [w10680] -> w10677
            shift-left: dbl[] [] -> [w10681]
            i -> [w10684]
            n4112 = case shown="13" w10684 {
              tunnel: w10683 -> [w10685 w10696 w10707 w10717 w10727 w10737 w10749 w10761 w10773 w10785 w10797 w10809 w10823 w10844 w10857 w10866 w10875]
              tunnel: [w10686 w10697 w10708 w10718 w10728 w10739 w10751 w10763 w10775 w10787 w10799 w10810 w10832 w10847 w10856 w10865 w10877] -> w10682
              frame 0, Default {
                # "总电压过高"
                n4113 = disable-structure shown="启用" {
                  disable-tunnel: [w10692 w10695] -> w10688
                  disable-tunnel: [w10691 w10695] -> w10687
                  disable-tunnel: w10685 -> [w10690 _]
                  frame Disabled {
                    n4114 = Unbundle By Name(w10690) -> ("总电压过高"=w10689:dbl)
                    n4115 = call "输入分辨率计算-EV05.vi"("1字节?"=FALSE, "数值"=w10689, "分辨率"=0.1) -> ("低字节"=w10692:dbl, "高字节1"=w10691:dbl)  [unwired: 2 in, 5 out]
                  }
                  frame Enabled {
                    w10695 = 255 ("高字节1")
                  }
                }
                n4116 = Build Array(w10687, w10688) -> (w10686:i32[])
              }
              frame 1 {
                # "总电压过低"
                n4117 = disable-structure shown="启用" {
                  disable-tunnel: [w10703 w10706] -> w10699
                  disable-tunnel: [w10702 w10706] -> w10698
                  disable-tunnel: w10696 -> [w10701 _]
                  frame Disabled {
                    n4118 = Unbundle By Name(w10701) -> ("总电压过低"=w10700:dbl)
                    n4119 = call "输入分辨率计算-EV05.vi"("1字节?"=FALSE, "数值"=w10700, "分辨率"=0.1) -> ("低字节"=w10703:dbl, "高字节1"=w10702:dbl)  [unwired: 2 in, 5 out]
                  }
                  frame Enabled {
                    w10706 = 255 ("高字节1")
                  }
                }
                n4120 = Build Array(w10698, w10699) -> (w10697:i32[])
              }
              frame 2 {
                # "温度过高"
                n4121 = disable-structure shown="启用" {
                  disable-tunnel: [w10713 255 ("高字节1")] -> w10709
                  disable-tunnel: w10707 -> [w10711 _]
                  frame Disabled {
                    n4122 = Unbundle By Name(w10711) -> ("温度过高"=w10710:dbl)
                    n4123 = call "输入分辨率计算-EV05.vi"("1字节?"=TRUE, "数值"=w10710, "偏移量"=-40.0, "分辨率"=1.0) -> ("高字节1"=w10713:dbl)  [unwired: 1 in, 6 out]
                  }
                  frame Enabled {
                  }
                }
                n4124 = Build Array(w10709) -> (w10708:i32[])
              }
              frame 3 {
                # "温度过低"
                n4125 = disable-structure shown="启用" {
                  disable-tunnel: [w10723 255 ("高字节1")] -> w10719
                  disable-tunnel: w10717 -> [w10721 _]
                  frame Disabled {
                    n4126 = Unbundle By Name(w10721) -> ("温度过低"=w10720:dbl)
                    n4127 = call "输入分辨率计算-EV05.vi"("1字节?"=TRUE, "数值"=w10720, "偏移量"=-40.0, "分辨率"=1.0) -> ("高字节1"=w10723:dbl)  [unwired: 1 in, 6 out]
                  }
                  frame Enabled {
                  }
                }
                n4128 = Build Array(w10719) -> (w10718:i32[])
              }
              frame 4 {
                # "整组温度不均衡"
                n4129 = disable-structure shown="启用" {
                  disable-tunnel: [w10733 255 ("高字节1")] -> w10729
                  disable-tunnel: w10727 -> [w10731 _]
                  frame Disabled {
                    n4130 = Unbundle By Name(w10731) -> ("整组温度不均衡"=w10730:dbl)
                    n4131 = call "输入分辨率计算-EV05.vi"("1字节?"=TRUE, "数值"=w10730, "偏移量"=0.0, "分辨率"=1.0) -> ("高字节1"=w10733:dbl)  [unwired: 1 in, 6 out]
                  }
                  frame Enabled {
                  }
                }
                n4132 = Build Array(w10729) -> (w10728:i32[])
              }
              frame 5 {
                # "单组电压不均衡"
                n4133 = disable-structure shown="启用" {
                  disable-tunnel: [w10745 w10748] -> w10740
                  disable-tunnel: [w10743 w10748] -> w10738
                  disable-tunnel: w10737 -> [w10742 _]
                  frame Disabled {
                    n4134 = Unbundle By Name(w10742) -> ("单组电压不均衡"=w10741:dbl)
                    n4135 = call "输入分辨率计算-EV05.vi"("1字节?"=FALSE, "数值"=w10741, "偏移量"=0.0, "分辨率"=0.001) -> ("低字节"=w10743:dbl, "高字节1"=w10745:dbl)  [unwired: 1 in, 5 out]
                  }
                  frame Enabled {
                    w10748 = 255 ("高字节1")
                  }
                }
                n4136 = Build Array(w10740, w10738) -> (w10739:i32[])
              }
              frame 6 {
                # "整组电压不均衡"
                n4137 = disable-structure shown="启用" {
                  disable-tunnel: [w10757 w10760] -> w10752
                  disable-tunnel: [w10755 w10760] -> w10750
                  disable-tunnel: w10749 -> [w10754 _]
                  frame Disabled {
                    n4138 = Unbundle By Name(w10754) -> ("整组电压不均衡"=w10753:dbl)
